vi "daqmx_linear_voltage_2ch.vi"() -> ()   [LabVIEW 2019]
uses:
  <vilib>/DAQmx/create/channels.llb/DAQmx Create Channel (AI-Voltage-Basic).vi
  <vilib>/DAQmx/configure/timing.llb/DAQmx Timing (Sample Clock).vi
  <vilib>/DAQmx/configure/task.llb/DAQmx Configure Logging (TDMS).vi
panel:
  out "data":waveform(dbl)[](array[waveform])=[{"t0"=timestamp(3655740824.5845337 s since 1904-01-01), "dt"=0.001, "Y"=[-0.8985024, -0.8902924, -0.882575, -0.8814256, -0.8814256, -0.8822466, -0.8819182, -0.881754, -0.8820824, -0.8824108], "attributes"=variant("NI_ChannelName"=variant(string "cDAQ1Mod1/ai0"), "NI_UnitDescription"=variant(string "Volts"))}, {"t0"=timestamp(3655740824.5845475 s since 1904-01-01), "dt"=0.001, "Y"=[-0.87026, -0.8778132000000001, -0.880112, -0.8809330000000001, -0.8814256, -0.8819182, -0.8815898000000001, -0.8814256, -0.8819182, -0.8822466], "attributes"=variant("NI_ChannelName"=variant(string "cDAQ1Mod1/ai1"), "NI_UnitDescription"=variant(string "Volts"))}]
  in  "NI-9205":tag="cDAQ1Mod1/ai0:1"
  out "Error Out":errorcluster
  in  "TDMS File":path=path "C:/Python/projects/nitdms/tests/tdms_files/daqmx_linear_voltage_2ch.tdms"
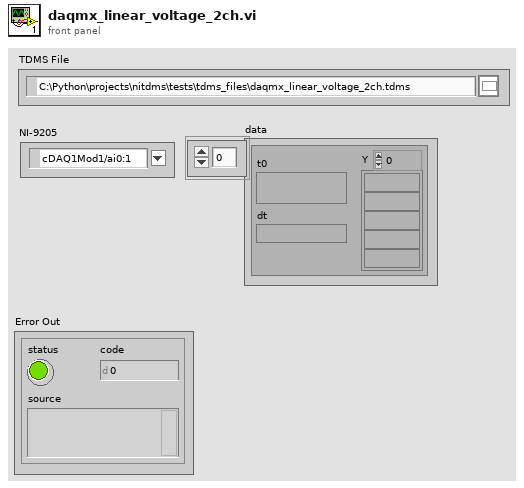
[diagram p1: front panel]
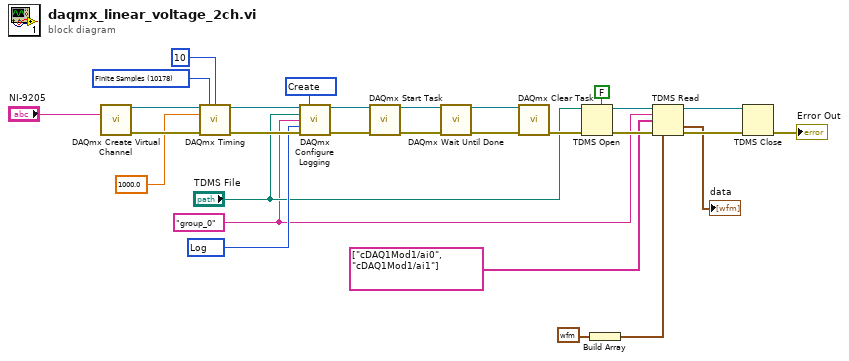
[diagram p0: block diagram]
diagram:
  w20 = 10178 items=["Finite Samples"=10178, "Continuous Samples"=10123, "Hardware Timed Single Point"=12522] ("sample mode")
  w23 = 15844 items=["Off"=10231, "Log"=15844, "Log and Read"=15842] ("logging mode")
  w9 = "group_0" ("group name")
  w24 = 15848 items=["Open"=10437, "Open or Create"=15846, "Create or Replace"=15847, "Create"=15848] ("operation")
  n1 = call-poly <vilib>:"DAQmx Create Virtual Channel.vi"("physical channels"="NI-9205") -> ("task out"=w28:refnum<k21>, "error out"=w29:errorcluster)  [unwired: 13 in]
  n2 = call-poly <vilib>:"DAQmx Timing.vi"("task/channels in"=w28, "sample mode"=w20, "samples per channel"=10, "rate"=1000.0, "error in"=w29) -> ("task out"=w25:refnum<k21>, "error out"=w26:errorcluster)  [unwired: 9 in]
  n3 = call-poly <vilib>:"DAQmx Configure Logging.vi"("task/channels in"=w25, "operation"=w24, "file path"="TDMS File", "group name"=w9, "logging mode"=w23, "error in"=w26) -> ("task out"=w21:refnum<k21>, "error out"=w22:errorcluster)  [unwired: 8 in]
  n4 = call <vilib>:"DAQmx Start Task.vi"("task/channels in"=w21, "error in"=w22) -> ("task out"=w17:refnum<k21>, "error out"=w18:errorcluster)  [unwired: 12 in]
  n5 = call <vilib>:"DAQmx Wait Until Done.vi"("task/channels in"=w17, "error in"=w18) -> ("task out"=w15:refnum<k21>, "error out"=w16:errorcluster)  [unwired: 12 in]
  n6 = call <vilib>:"DAQmx Clear Task.vi"("task in"=w15, "error in"=w16) -> ("error out"=w14:errorcluster)  [unwired: 13 in]
  n7 = TDMS Open(5:FALSE ("create index file? (T)"), 8:w14, 11:"TDMS File") -> (0:w11:errorcluster, 3:w10:refnum<k34>)  [unwired: 4 in]
  n8 = Build Array(waveform(dbl) {"t0"=timestamp(0 s since 1904-01-01), "dt"=1.0, "Y"=[]} ("Waveform")) -> (w2:waveform(dbl)[])
  n9 = TDMS Read(0:w10, 5:w9, 7:string[] ["cDAQ1Mod1/ai0", "cDAQ1Mod1/ai1"], 11:w11, 12:w2) -> (4:w6:refnum<k34>, 10:→"data":waveform(dbl)[], 15:w7:errorcluster)  [unwired: 3 in, 3 out]
  n10 = TDMS Close(8:w7, 11:w6) -> (0:→"Error Out":errorcluster)  [unwired: 1 out]
